vi "LED-Facade.vi"(0 "Data In":T4, 2 "Display State In":T2, 3 "Container State":T3) -> (6 "Data Out":T4, 7 "Display State Out":T2, 8 "Action":T1)   [LabVIEW 2010, in "LED Display.xctl"]
uses:
  LED Display.xctl
  LED-Data.ctl
  <vilib>/_xctls/Container State.ctl
  LED-State.ctl
  <vilib>/_xctls/Action.ctl
  <vilib>/_xctls/XControlSupport.lvlib
panel:
  out "LED Display":bool[][](array[boolean])
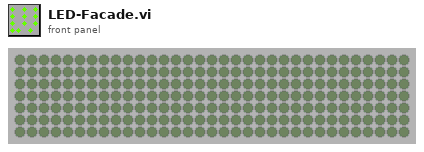
[diagram p1: front panel]
types:
  T1 = typedef "XControlSupport.lvlib/Action.ctl" = cluster{"Data Changed?":bool, "State Changed?":bool, "Action Name":string}
  T2 = typedef "LED Display.xctl/LED-State.ctl" = cluster{"Flags":u64}
  T3 = typedef "XControlSupport.lvlib/Container State.ctl" = cluster{"Indicator?":bool, "Run Mode?":bool, " Refnum":refnum<vi>}
  T4 = typedef "LED Display.xctl/LED-Data.ctl" = string
  T5 = typedef "LVRectTypeDef.ctl" = cluster{"left":i16, "top":i16, "right":i16, "bottom":i16}
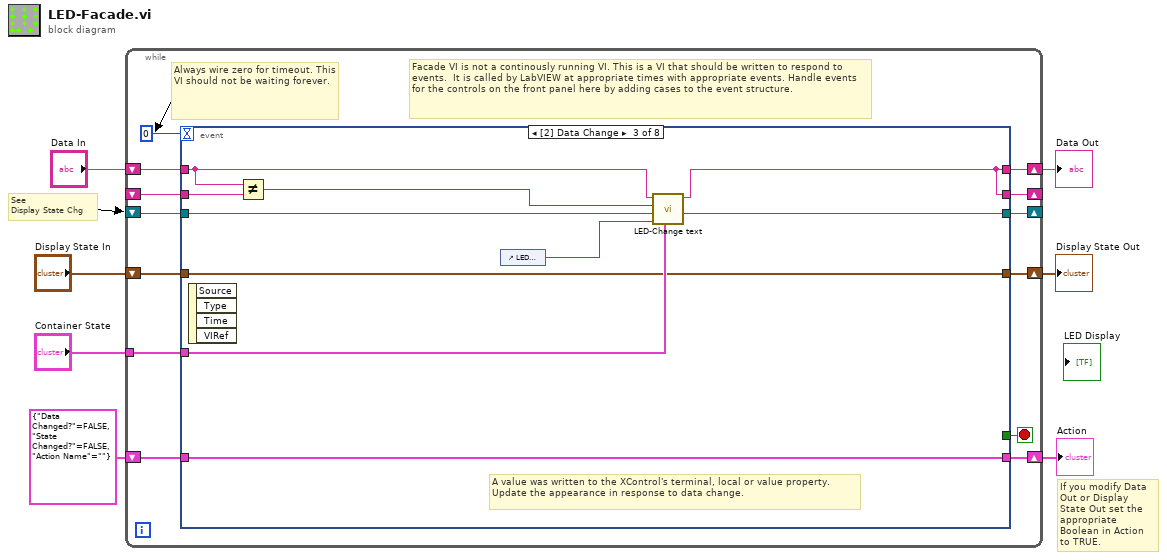
[diagram p0: block diagram]
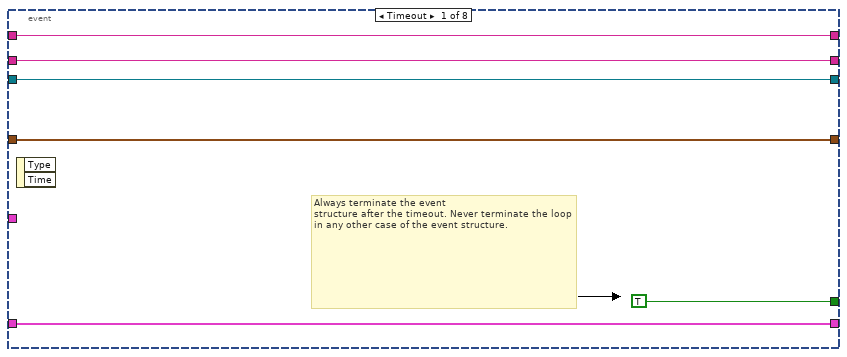
[diagram p2: hidden frame]
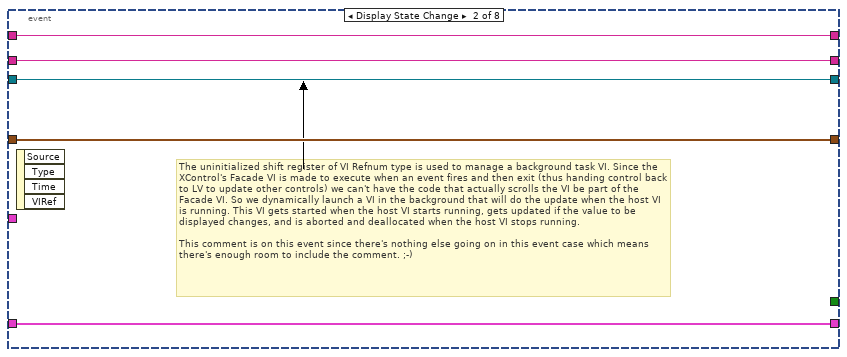
[diagram p3: hidden frame]
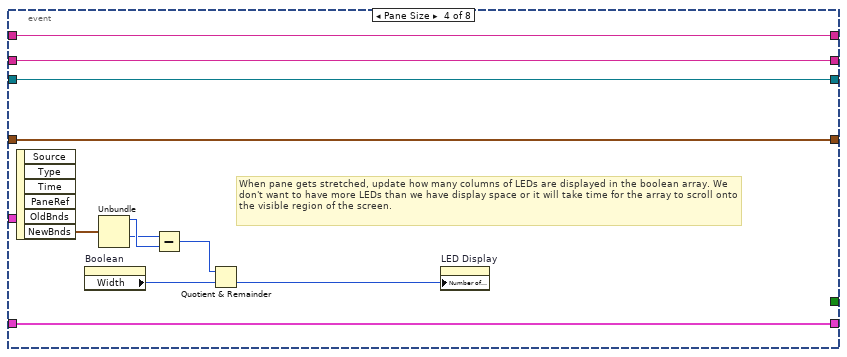
[diagram p4: hidden frame]
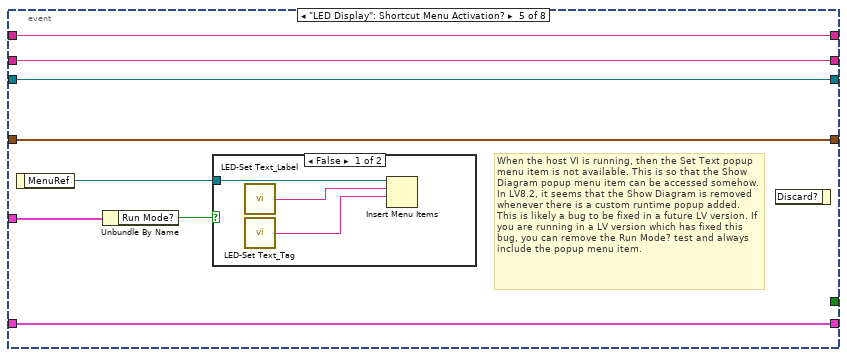
[diagram p5: hidden frame]
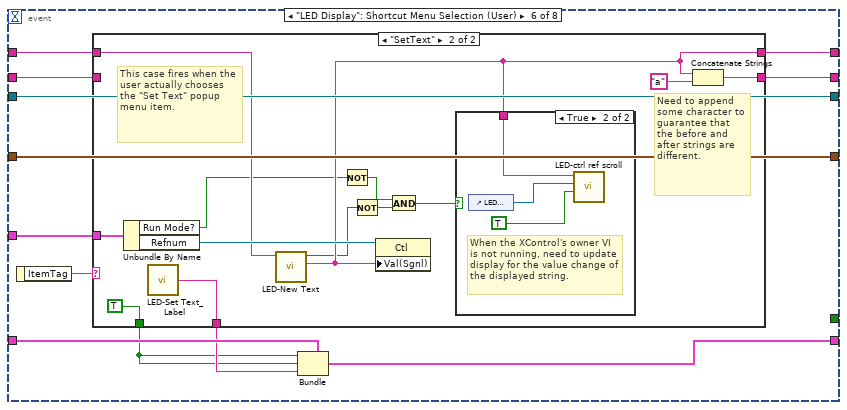
[diagram p7: hidden frame]
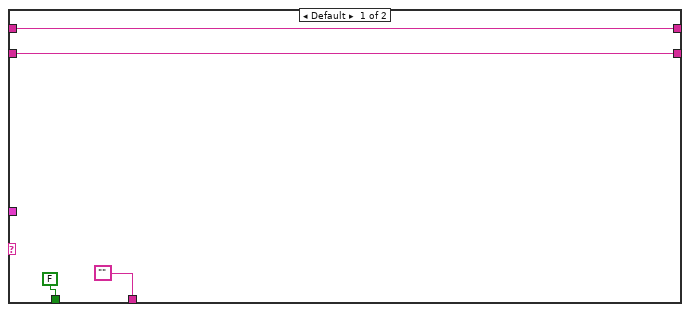
[diagram p8: hidden frame]
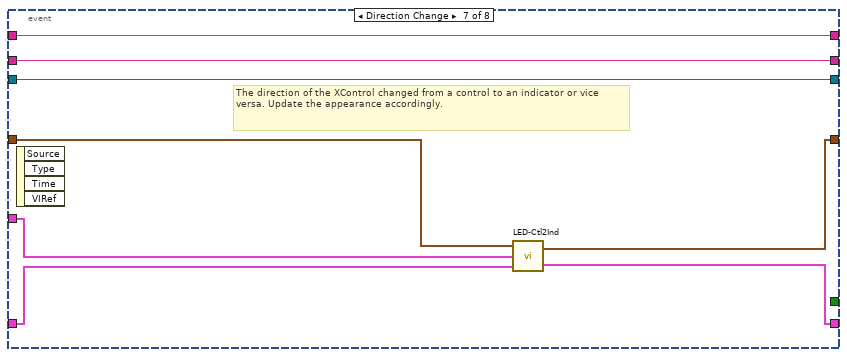
[diagram p10: hidden frame]
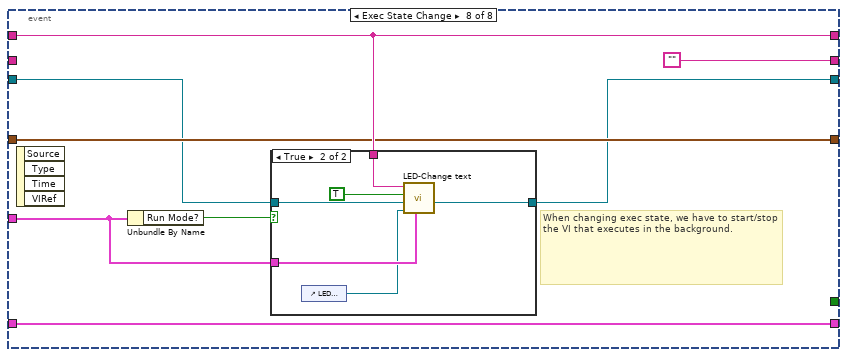
[diagram p11: hidden frame]
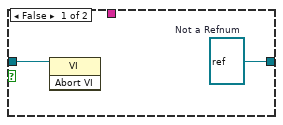
[diagram p12: hidden frame]
diagram:
  # "See\nDisplay State Chg"
  # "If you modify Data Out or Display State Out set the appropriate Boolean in Action to TRUE."
  n1 = while {
    shift-right: [w19] -> w4
    shift-left: "Display State In" -> [w20]
    tunnel: "Container State" -> [w16]
    shift-right: [w14] -> w7
    shift-left: "Data In" -> [w15]
    shift-right: [w12] -> w2
    shift-left: T1 {"Data Changed?"=FALSE, "State Changed?"=FALSE, "Action Name"=""} ("Action") -> [w13]
    shift-right: [w11] -> _
    shift-left: _ -> [w10]
    shift-right: [w9] -> _
    shift-left: _ -> [w8]
    stop <- w18 stop-if-true
    # "Facade VI is not a continously running VI. This is a VI that should be written to respond to events.  It is called by LabVIEW at appropriate times with appropriate events. Handle events for the controls on the front panel here by adding cases to the event structure."
    # "Always wire zero for timeout. This\nVI should not be waiting forever."
    n2 = event shown="[2] Data Change" {
      selector: _ -> [_ _ _ _ _ _ _ _]
      dyn-events: _ -> [_ _ _ _ _ _ _ _]
      timeout: 0 -> [_ _ _ _ _ _ _ _]
      tunnel: w20 -> [w24 w31 w32 w50 w57 w73 w100 w106]
      tunnel: [w24 w31 w32 w50 w57 w73 w99 w106] -> w19
      tunnel: [TRUE _ _ _ _ _ _ _] -> w18
      tunnel: w16 -> [_ _ w41 _ w59 w65 w102 w108]
      tunnel: w15 -> [w23 w29 w36 w52 w55 w69 w103 w109]
      tunnel: [w23 w29 w37 w52 w55 w71 w103 w109] -> w14
      tunnel: [w25 w30 w35 w49 w54 w74 w97 w107] -> w12
      tunnel: w13 -> [w25 w30 w35 w49 w54 w75 w98 w107]
      tunnel: [w22 w28 w37 w51 w56 w72 w101 ""] -> w11
      tunnel: w10 -> [w22 w28 w40 w51 w56 w68 w101 _]
      tunnel: [w21 w27 w34 w44 w53 w64 w96 w105] -> w9
      tunnel: w8 -> [w21 w27 w33 w44 w53 w64 w96 w104]
      event Timeout {
        # "Always terminate the event\nstructure after the timeout. Never terminate the loop in any other case of the event structure."
        n3 = event-data() -> ()  [unwired: 1 in, 2 out]
      }
      event Display State Change {
        # "The uninitialized shift register of VI Refnum type is used to manage a background task VI. Since the XControl's Facade VI is made to execute when an event fires and then exit (thus handing control back to LV to update other controls) we can't have the code that actually scrolls the VI be part of the Facade VI. So we dynamically launch a VI in the background that will do the update when the host VI is running. This VI gets started when the host VI starts running, gets updated if the value to be displayed changes, and is aborted and deallocated when the host VI stops running.\n\nThis comment is on this event since there's nothing else going on in this event case which means there's enough room to include the comment. ;-)"
        n4 = event-data() -> ()  [unwired: 1 in, 4 out]
      }
      event Data Change {
        # "A value was written to the XControl's terminal, local or value property.\nUpdate the appearance in response to data change."
        n5 = event-data() -> ()  [unwired: 1 in, 4 out]
        n6 = Not Equal?(x=w36, y=w40) -> (x != y?=w39:bool)
        n7 = control-ref of="LED Display"() -> (w38:refnum<vi>)
        n8 = call "LED-Change text.vi"("Container State"=w41, "LED Display"=w38, "vi reference in"=w33, "Should Change?"=w39, "Data In"=w36) -> ("vi reference out"=w34:refnum<vi>, "Data Out"=w37:T4)  [unwired: 3 in]
      }
      event Pane Size {
        # "When pane gets stretched, update how many columns of LEDs are displayed in the boolean array. We don't want to have more LEDs than we have display space or it will take time for the array to scroll onto the visible region of the screen."
        n9 = event-data() -> ("NewBnds"=w48:T5)  [unwired: 1 in, 5 out]
        n10 = property on="Boolean" class="Bool (strict)"() -> ("Width"=w42:u32)  [unwired: 2 in, 2 out]
        n11 = Unbundle(w48) -> ("left"=w46:i16, "right"=w45:i16)  [unwired: 2 out]
        n12 = Subtract(x=w45, y=w46) -> (x-y=w47:i16)
        n13 = Quotient & Remainder(x=w47, y=w42) -> (floor(x/y)=w43:u32)  [unwired: 1 out]
        n14 = property on="LED Display" class="Arr (strict)"("Number of Columns"=w43) -> ()  [unwired: 2 in, 2 out]
      }
      event "LED Display": Shortcut Menu Activation? {
        # "When the host VI is running, then the Set Text popup menu item is not available. This is so that the Show Diagram popup menu item can be accessed somehow. In LV8.2, it seems that the Show Diagram is removed whenever there is a custom runtime popup added. This is likely a bug to be fixed in a future LV version. If you are running in a LV version which has fixed this bug, you can remove the Run Mode? test and always include the popup menu item."
        n15 = event-data() -> ("MenuRef"=w60:refnum<k9>)  [unwired: 1 in]
        n16 = Unbundle By Name(w59) -> ("Run Mode?"=w58:bool)
        n17 = case shown="False" w58 {
          tunnel: w60 -> [w63 _]
          frame False {
            n18 = call "LED-Set Text_Label.vi"() -> ("\"Set Text\" Label"=w62:string)
            n19 = call "LED-Set Text_Tag.vi"() -> ("\"Set Text\" Label"=w61:string)
            n20 = Insert Menu Items(7:w61, 8:w62, 9:w63) -> ()  [unwired: 3 in, 3 out]
          }
          frame True {
          }
        }
        n21 = event-data() -> ()  [unwired: 2 in, 1 out]
      }
      event "LED Display": Shortcut Menu Selection (User) {
        n22 = event-data() -> ("ItemTag"=w70:string)  [unwired: 1 in]
        n23 = case shown="\"SetText\"" w70 {
          tunnel: [w78 w91] -> w72
          tunnel: [w79 w85] -> w71
          tunnel: [FALSE TRUE] -> w66
          tunnel: w69 -> [w79 w86]
          tunnel: w68 -> [w78 _]
          tunnel: ["" w89] -> w67
          tunnel: w65 -> [_ w88]
          frame Default {
          }
          frame "SetText" {
            # "This case fires when the user actually chooses the \"Set Text\" popup menu item."
            # "Need to append some character to guarantee that the before and after strings are different."
            n24 = Unbundle By Name(w88) -> ("Run Mode?"=w84:bool, "Refnum"=w87:refnum<vi>)
            n25 = call "LED-Set Text_Label.vi"() -> ("\"Set Text\" Label"=w89:string)
            n26 = call "LED-New Text.vi"("Current Text"=w86) -> ("New text"=w85:string, "Cancelled?"=w81:bool)  [unwired: 9 in]
            n27 = Not(x=w84) -> (.not. x?=w83:bool)
            n28 = Not(x=w81) -> (.not. x?=w82:bool)
            n29 = property class="Ctl"(reference=w87, "Val(Sgnl)"=w85) -> ()  [unwired: 1 in, 2 out]
            n30 = And(x=w83, y=w82) -> (x .and. y?=w80:bool)
            n31 = case shown="True" w80 {
              tunnel: w85 -> [_ w95]
              frame False {
              }
              frame True {
                # "When the XControl's owner VI\nis not running, need to update\ndisplay for the value change of\nthe displayed string."
                n32 = control-ref of="LED Display"() -> (w94:refnum<vi>)
                n33 = call "LED-ctrl ref scroll.vi"("Single pass?"=TRUE, "LEDDisplay"=w94, "String"=w95) -> ()  [unwired: 9 in]
              }
            }
            n34 = Concatenate Strings(w85, "a" ("string")) -> (w91:string)
          }
        }
        n35 = Bundle(cluster=w75, "Data Changed?"=w66, "State Changed?"=w66, "Action Name"=w67) -> (w74:T1)
      }
      event Direction Change {
        # "The direction of the XControl changed from a control to an indicator or vice versa. Update the appearance accordingly."
        n36 = event-data() -> ()  [unwired: 1 in, 4 out]
        n37 = call "LED-Ctl2Ind.vi"("Action 2"=w98, "Container State"=w102, "Display State In 2"=w100) -> ("Action"=w97:T1, "Display State In"=w99:T2)
      }
      event Exec State Change {
        # "When changing exec state, we have to start/stop the VI that executes in the background."
        n38 = event-data() -> ()  [unwired: 1 in, 4 out]
        n39 = Unbundle By Name(w108) -> ("Run Mode?"=w111:bool)
        n40 = case shown="True" w111 {
          tunnel: [w113 w115] -> w105
          tunnel: w109 -> [_ w119]
          tunnel: w108 -> [_ w117]
          tunnel: w104 -> [w112 w114]
          frame False {
            w113 = refnum<vi> refnum  # Not a Refnum
            n41 = invoke class="VI" method="Abort VI"(reference=w112) -> ()  [unwired: 2 in, 3 out]
          }
          frame True {
            n42 = control-ref of="LED Display"() -> (w116:refnum<vi>)
            n43 = call "LED-Change text.vi"("Container State"=w117, "LED Display"=w116, "vi reference in"=w114, "Should Change?"=TRUE, "Data In"=w119) -> ("vi reference out"=w115:refnum<vi>)  [unwired: 3 in, 1 out]
          }
        }
      }
    }
  }
  "Display State Out" <- w4
  "Data Out" <- w7
  "Action" <- w2
